vi "Practica 3 - Combinacion de operaciones.vi"() -> ()   [LabVIEW 2023]
panel:
  out "DIVISION":dbl
  out "MULTIPLICACION":dbl
  out "RESTA":dbl
  out "SUMA":dbl
  in  "Z":dbl
  in  "Y":dbl
  in  "X":dbl
  # "OPERACIONES BASICAS"
  # "Datos de entrada"
  # "Resultado"
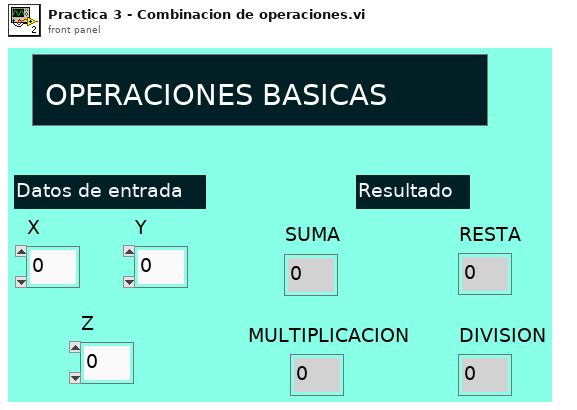
[diagram p1: front panel]
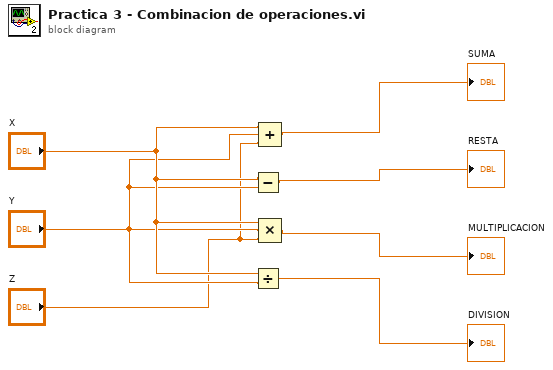
[diagram p0: block diagram]
diagram:
  n1 = Subtract(x="X", y="Y") -> (x-y=→"RESTA":dbl)
  n2 = Divide(x="X", y="Y") -> (x/y=→"DIVISION":dbl)
  n3 = Compound Arithmetic op=ADD("X", "Y", "Z") -> (→"SUMA":dbl)
  n4 = Compound Arithmetic op=MULTIPLY("X", "Y", "Z") -> (→"MULTIPLICACION":dbl)
